vi "selectStepTrigger.vi"(3 "stepTriggerEdge":T1=enum."true-false", 4 "MCSSelectStepTrigger":T2, 5 "triggerReadout":u16) -> (1 "fired":bool)   [LabVIEW 2014]
uses:
  Controls/selectTrigger.ctl
  Controls/triggerEdge.ctl
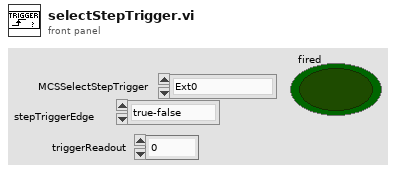
[diagram p1: front panel]
types:
  T1 = typedef "triggerEdge.ctl" = enum8{"either", "false-true", "true-false"}
  T2 = typedef "selectTrigger.ctl" = enum8{"Ext0", "Ext1", "Ext2", "Ext3", "Ext4", "Ext5", "Ext6", "Ext7", "Int0", "Int1", "Int2", "Int3", "Int4", "Int5", "Int6", "Int7"}
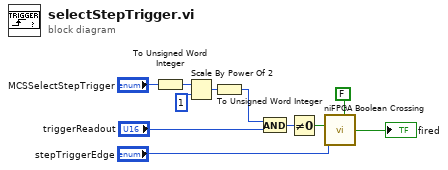
[diagram p0: block diagram]
diagram:
  n1 = To Unsigned Word Integer(number="MCSSelectStepTrigger") -> (unsigned 16bit integer=w6:u16)
  n2 = Scale By Power Of 2(n=w6, x=i16 1) -> (x*2^n=w4:i16)
  n3 = To Unsigned Word Integer(number=w4) -> (unsigned 16bit integer=w3:u16)
  n4 = And(x=w3, y="triggerReadout") -> (x .and. y?=w7:u16)
  n5 = Not Equal To 0?(x=w7) -> (x != 0?=w2:bool)
  n6 = call <vilib>:"niFPGA Boolean Crossing.vi"("input"=w2, "direction"="stepTriggerEdge", "initialize"=FALSE) -> ("crossing"=→"fired":bool)  [unwired: 6 in]
